vi "test_CCDAcquisitionSequence.vi"(7 "Test should pass":bool=TRUE, 8 "error in":errorcluster, 9 "tear down connection":bool=TRUE, 10 "set-up a connection":bool=TRUE, 11 "device selection":enum16{"monochromator", "CCD", "SCD"}(ring)=enum."CCD") -> (0 "error out":errorcluster)   [LabVIEW 2023]
uses:
  Classes/CCD/CCD.lvclass
  C:/Projects/Horiba/horiba-labview-sdk/Source/Classes/GenericDevice/GenericDevice.lvclass
  <vilib>/addons/_JKI Toolkits/Caraya/classes/Assert/Assert Equal Value and Type_Variant.vi
  <vilib>/addons/_JKI Toolkits/Caraya/classes/Assert/Assert Not Error.vi
  <vilib>/addons/_JKI Toolkits/Caraya/classes/Test/Test.lvclass
  <vilib>/addons/_JKI Toolkits/Caraya/classes/Assert/Assert.lvclass
panel:
  out "results-JSON string":string
  # "Connector Pane"
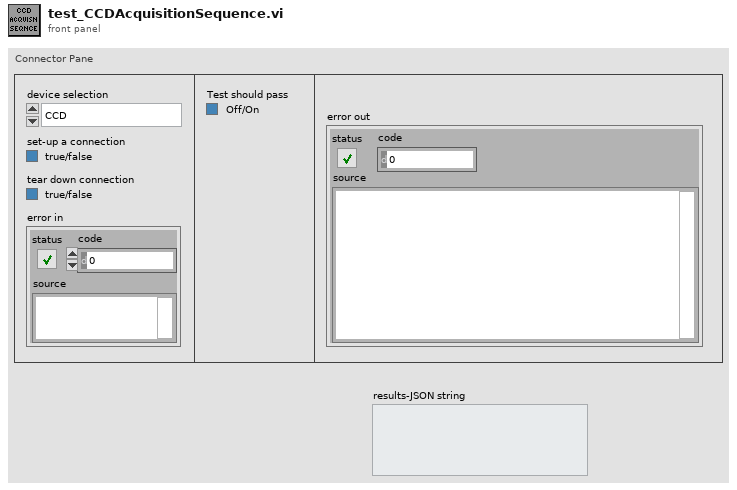
[diagram p1: front panel]
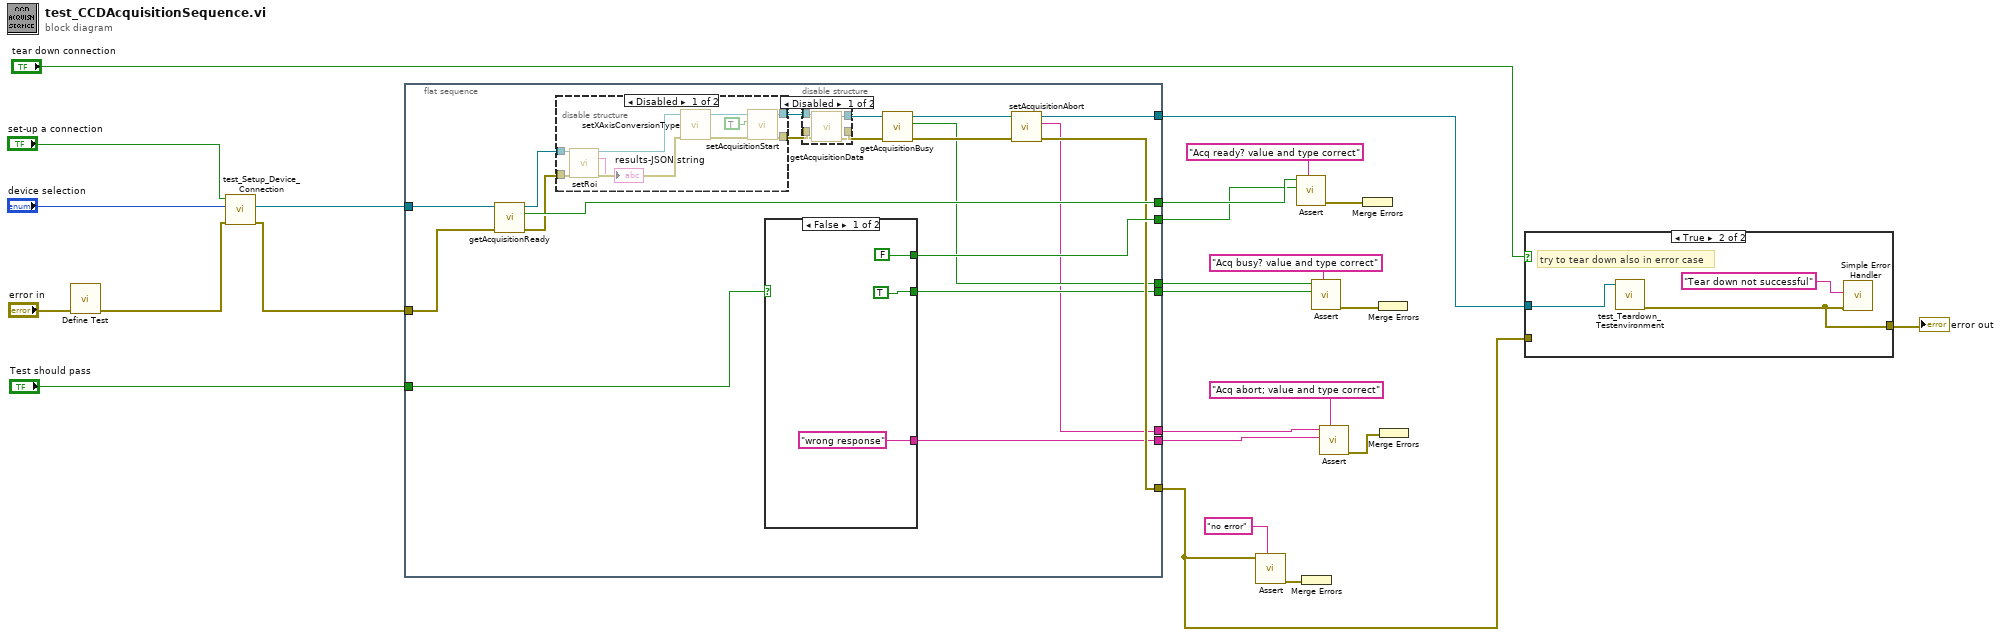
[diagram p0: block diagram]
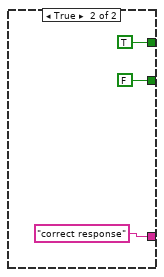
[diagram p4: hidden frame]
diagram:
  n1 = call <vilib>:"Define Test.vi"("error in (no error)"="error in") -> ("error out"=w11:errorcluster)  [unwired: 9 in, 1 out]
  n2 = call "test_Setup_Device_Connection.vi"("error in (no error)"=w11, "device selection"="device selection", "set-up a connection"="set-up a connection") -> ("error out"=w12:errorcluster, "CCD out"=w13:refnum<class "CCD.lvclass">)  [unwired: 5 in, 2 out]
  n3 = flat-sequence {
    tunnel: [w43] -> w23
    tunnel: w12 -> [w31]
    tunnel: w13 -> [w32]
    tunnel: [w36] -> w17
    tunnel: "Test should pass" -> [w44]
    tunnel: [w37] -> w16
    tunnel: [w42] -> w14
    tunnel: [w29] -> w6
    tunnel: [w28] -> w5
    tunnel: [w27] -> w2
    tunnel: [w26] -> w1
    frame #0 {
      n4 = call "getAcquisitionReady.vi"("error in (no error)"=w31, "CCD in"=w32) -> ("error out"=w38:errorcluster, "ready"=w43:bool, "CCD out"=w41:refnum<class "CCD.lvclass">)  [unwired: 7 in]
      n5 = disable-structure shown="Disabled" {
        disable-tunnel: w41 -> [w54 _]
        disable-tunnel: [w49 _] -> w40
        disable-tunnel: [w48 _] -> w39
        disable-tunnel: w38 -> [w47 _]
        frame Disabled {
          n6 = call "setRoi.vi"("CCD in"=w54, "error in (no error)"=w47) -> ("CCD out"=w53:refnum<class "CCD.lvclass">, "results-JSON string"=→"results-JSON string":string, "error out"=w52:errorcluster)  [unwired: 10 in, 1 out]
          n7 = call "setXAxisConversionType.vi"("error in (no error)"=w52, "CCD in"=w53) -> ("error out"=w50:errorcluster, "CCD out"=w51:refnum<class "CCD.lvclass">)  [unwired: 6 in, 2 out]
          n8 = call "setAcquisitionStart.vi"("error in (no error)"=w50, "openShutter"=TRUE, "CCD in"=w51) -> ("error out"=w48:errorcluster, "CCD out"=w49:refnum<class "CCD.lvclass">)  [unwired: 5 in, 2 out]
        }
        frame Enabled {
        }
      }
      n9 = case shown="False" w44 {
        tunnel: [FALSE TRUE] -> w42
        tunnel: [TRUE FALSE] -> w28
        tunnel: ["wrong response" "correct response"] -> w26
        frame False {
        }
        frame True {
        }
      }
      n10 = disable-structure shown="Disabled" {
        disable-tunnel: w40 -> [w58 _]
        disable-tunnel: w39 -> [w57 _]
        disable-tunnel: [w56 _] -> w34
        disable-tunnel: [w55 _] -> w35
        frame Disabled {
          n11 = call "getAcquisitionData.vi"("error in (no error)"=w57, "CCD in"=w58) -> ("error out"=w55:errorcluster, "CCD out"=w56:refnum<class "CCD.lvclass">)  [unwired: 8 in]
        }
        frame Enabled {
        }
      }
      n12 = call "getAcquisitionBusy.vi"("error in (no error)"=w35, "CCD in"=w34) -> ("error out"=w30:errorcluster, "isBusy"=w29:bool, "CCD out"=w33:refnum<class "CCD.lvclass">)  [unwired: 7 in]
      n13 = call "setAcquisitionAbort.vi"("error in (no error)"=w30, "CCD in"=w33) -> ("error out"=w36:errorcluster, "results-JSON string"=w27:string, "CCD out"=w37:refnum<class "CCD.lvclass">)  [unwired: 6 in, 1 out]
    }
  }
  n14 = call-poly <vilib>:"Assert.vi"("Label"="no error" ("Label (VI Title)"), "Not Error?"=w17) -> ("error out"=w19:errorcluster)  [unwired: 8 in, 1 out]
  n15 = call-poly <vilib>:"Assert.vi"("Label"="Acq ready? value and type correct" ("Label (VI Title)"), "Y"=w14, "X"=w23) -> ("error out"=w24:errorcluster)  [unwired: 7 in, 1 out]
  n16 = Merge Errors(w19) -> ()  [unwired: 1 out]
  n17 = call-poly <vilib>:"Assert.vi"("Label"="Acq busy? value and type correct" ("Label (VI Title)"), "Y"=w5, "X"=w6) -> ("error out"=w8:errorcluster)  [unwired: 7 in, 1 out]
  n18 = call-poly <vilib>:"Assert.vi"("Label"="Acq abort; value and type correct" ("Label (VI Title)"), "Y"=w1, "X"=w2) -> ("error out"=w3:errorcluster)  [unwired: 7 in, 1 out]
  n19 = Merge Errors(w24) -> ()  [unwired: 1 out]
  n20 = Merge Errors(w8) -> ()  [unwired: 1 out]
  n21 = Merge Errors(w3) -> ()  [unwired: 1 out]
  n22 = case shown="True" "tear down connection" {
    tunnel: w16 -> [_ w67]
    tunnel: [w65 w66] -> w15
    tunnel: w17 -> [w65 _]
    frame False {
    }
    frame True {
      # "try to tear down also in error case"
      n23 = call "test_Teardown_Testenvironment.vi"("GenericDevice.lvclass"=w67) -> ("error out"=w66:errorcluster)  [unwired: 9 in, 1 out]
      n24 = call <vilib>:"Simple Error Handler.vi"("error source (\" \")"="Tear down not successful" ("error source (\" \")"), "error in (no error)"=w66) -> ()  [unwired: 3 in, 5 out]
    }
  }
  "error out" <- w15
